vi "Handle Error.vi"(8 "error in (no error)":errorcluster, 11 "MSS Target Actor in":refnum<class "MSS Target Actor.lvclass">) -> (0 "error out":errorcluster, 2 "stop actor?":bool=TRUE, 3 "MSS Target Actor out":refnum<class "MSS Target Actor.lvclass">)   [LabVIEW 2024, in "MSS Target Actor.lvlib" / "MSS Target Actor.lvclass"]
doc: "(<B>Filename</B>: Actor Framework.lvlib:Actor.lvclass:Handle Error.vi)\n\nDefines how the actor handles an error that occurred while processing a message. By default, this method does nothing except stop the actor."
uses:
  MSS Target Actor.lvclass
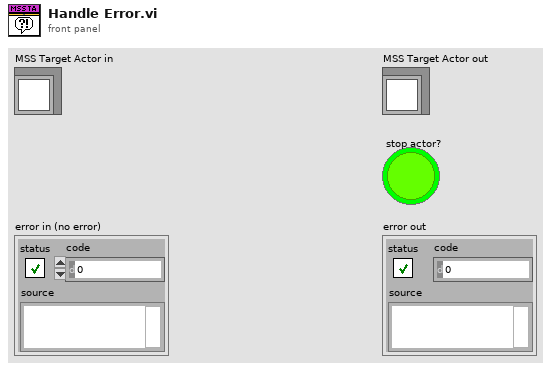
[diagram p1: front panel]
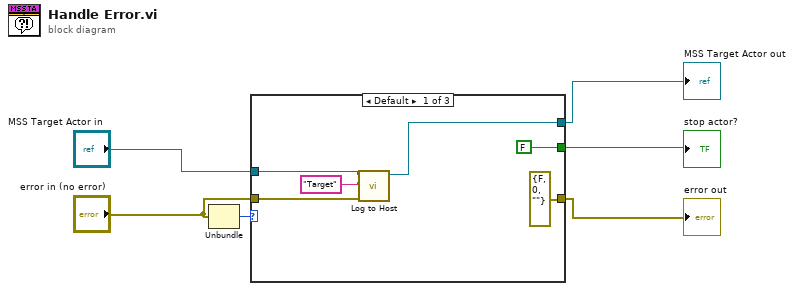
[diagram p0: block diagram]
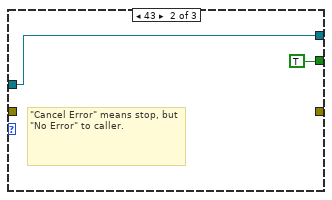
[diagram p2: hidden frame]
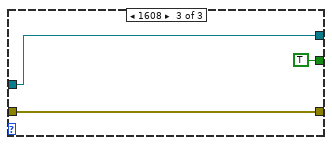
[diagram p3: hidden frame]
diagram:
  n1 = Unbundle("error in (no error)") -> ("code"=w6:i32)  [unwired: 2 out]
  n2 = case shown="Default" w6 {
    tunnel: [errorcluster {"status"=FALSE, "code"=0, "source"=""} ("error out") _ w16] -> w4
    tunnel: "error in (no error)" -> [w12 _ w16]
    tunnel: [FALSE ("stop actor?") TRUE ("stop actor?") TRUE ("stop actor?")] -> w3
    tunnel: "MSS Target Actor in" -> [w9 w14 w15]
    tunnel: [w8 w14 w15] -> w1
    frame Default {
      n3 = call "Log to Host.vi"("error in"=w12, "Detail"="Target", "MSS Target Actor in"=w9) -> ("MSS Target Actor out"=w8:refnum<class "MSS Target Actor.lvclass">)  [unwired: 7 in, 1 out]
    }
    frame 43 {
      # "\"Cancel Error\" means stop, but \"No Error\" to caller."
    }
    frame 1608 {
    }
  }
  "MSS Target Actor out" <- w1
  "error out" <- w4
  "stop actor?" <- w3
